vi "thermalCamera.vi"() -> ()   [LabVIEW 2025]
panel:
  in  "Stop Button":bool
  out "Output":string
  in  "Flag":bool
  in  "Stop recording":bool
  in  "Stop Preview":bool
  in  "Server Path":path
  in  "Focus":dbl(slide) scale=0.0..100.0
  in  "Record":bool
  in  "Connect Server":bool
  out "?":string
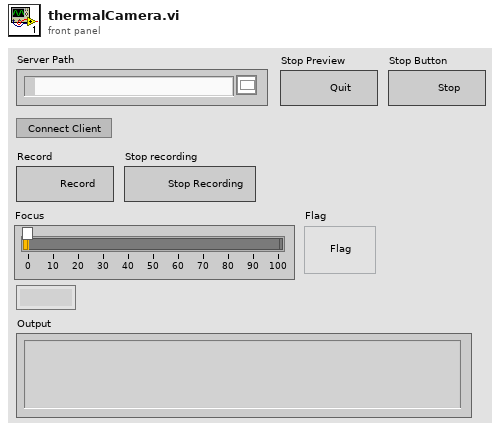
[diagram p1: front panel]
types:
  T1 = enum16{"Standard", "Buffered", "CRLF", "Immediate"}
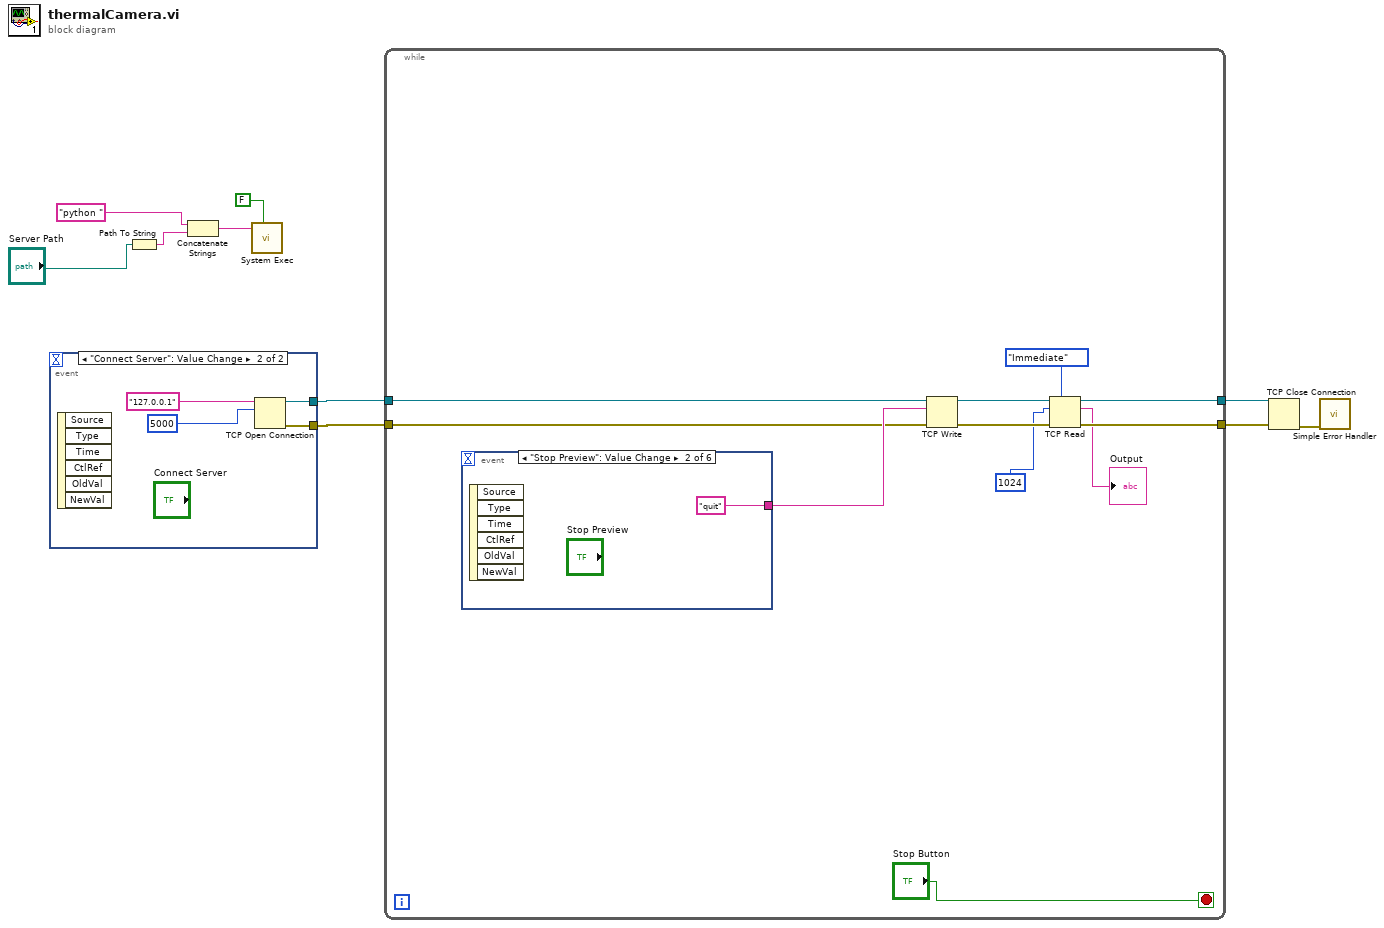
[diagram p0: block diagram]
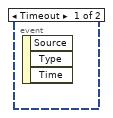
[diagram p2: hidden frame]
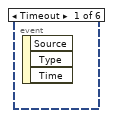
[diagram p3: hidden frame]
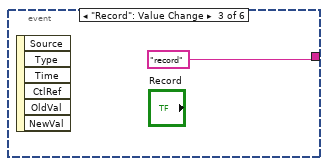
[diagram p4: hidden frame]
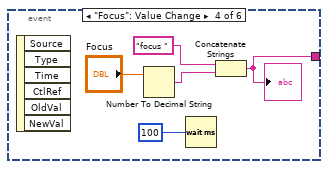
[diagram p5: hidden frame]
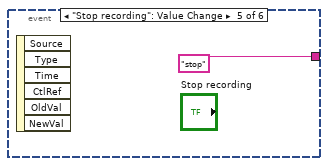
[diagram p6: hidden frame]
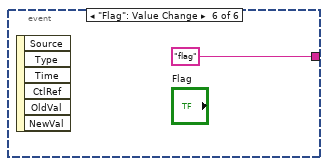
[diagram p7: hidden frame]
diagram:
  n1 = event shown="[1] \"Connect Server\": Value Change" {
    selector: _ -> [_ _]
    dyn-events: _ -> [_ _]
    timeout: _ -> [_ _]
    tunnel: [_ w12] -> w5
    tunnel: [_ w11] -> w4
    event Timeout {
      n2 = event-data() -> ()  [unwired: 1 in, 3 out]
    }
    event "Connect Server": Value Change {
      n3 = event-data() -> ()  [unwired: 1 in, 6 out]
      n4 = TCP Open Connection(address="127.0.0.1", remote port or service name=u16 5000) -> (connection ID=w11:refnum<k5>, error out=w12:errorcluster)  [unwired: 3 in]
    }
  }
  n5 = Path To String(path="Server Path") -> (string=w6:string)
  n6 = Concatenate Strings("python " ("string"), w6) -> (w2:string)
  n7 = call <vilib>:"System Exec.vi"("wait until completion? (T)"=FALSE, "command line"=w2) -> ()  [unwired: 6 in, 4 out]
  n8 = while {
    tunnel: [w24] -> w10
    tunnel: [w22] -> w9
    tunnel: w5 -> [w20]
    tunnel: w4 -> [w19]
    stop <- "Stop Button" stop-if-true
    n9 = event shown="[1] \"Stop Preview\": Value Change" {
      selector: _ -> [_ _ _ _ _ _]
      dyn-events: _ -> [_ _ _ _ _ _]
      timeout: _ -> [_ _ _ _ _ _]
      tunnel: [_ "quit" "record" w30 "stop" "flag"] -> w21
      event Timeout {
        n10 = event-data() -> ()  [unwired: 1 in, 3 out]
      }
      event "Stop Preview": Value Change {
        n11 = event-data() -> ()  [unwired: 1 in, 6 out]
      }
      event "Record": Value Change {
        n12 = event-data() -> ()  [unwired: 1 in, 6 out]
      }
      event "Focus": Value Change {
        n13 = event-data() -> ()  [unwired: 1 in, 6 out]
        n14 = Number To Decimal String(number="Focus") -> (decimal integer string=w32:string)  [unwired: 1 in]
        n15 = Wait (ms)(milliseconds to wait=u32 100) -> ()  [unwired: 1 out]
        n16 = Concatenate Strings("focus ", w32) -> (w30:string)
        "?" <- w30
      }
      event "Stop recording": Value Change {
        n17 = event-data() -> ()  [unwired: 1 in, 6 out]
      }
      event "Flag": Value Change {
        n18 = event-data() -> ()  [unwired: 1 in, 6 out]
      }
    }
    n19 = TCP Write(connection ID=w19, data in=w21, error in (no error)=w20) -> (connection ID out=w23:refnum<k5>, error out=w25:errorcluster)  [unwired: 1 in, 1 out]
    n20 = TCP Read(connection ID=w23, bytes to read=1024, error in (no error)=w25, 7:T1."Immediate" ("mode (standard)")) -> (connection ID out=w22:refnum<k5>, data out=→"Output":string, error out=w24:errorcluster)  [unwired: 1 in]
  }
  n21 = TCP Close Connection(connection ID=w9, error in (no error)=w10) -> (error out=w8:errorcluster)  [unwired: 1 in, 1 out]
  n22 = call <vilib>:"Simple Error Handler.vi"("error in (no error)"=w8) -> ()  [unwired: 4 in, 5 out]
